vi "main.vi"() -> ()   [LabVIEW 2021]
uses:
  Global 1.vi
panel:
  in  "Boolean 2":bool
  in  "Tab Control":T1(tab)
  out "Curvas luz y temperatura":cluster{"Ramp Pattern":dbl[], dbl[]}[](graph)
  in  "Load":bool
  in  "Export":bool
  in  "Curva de Luz":path
  in  "Curva de Temperatura":path
  in  "Ruta Luz":path
  in  "Ruta Temperatura":path
  in  "Integrate":bool
  in  "X1 (s)":dbl
  in  "X2 (s)":dbl
  out "Resultado":dbl
  in  "Load 2":bool
  in  "Load 3":bool
  out "Curvas  Luz":cluster{"Ramp Pattern":dbl[], u32[]}[](graph)
  in  "Luz 4":path
  in  "Luz 3":path
  in  "Luz 2":path
  in  "Luz 1":path
  in  "Temperatura 4":path
  in  "Temperatura 3":path
  in  "Temperatura 2":path
  in  "Temperatura 1":path
  out "Curvas Temperatura":cluster{"Ramp Pattern":dbl[], u32[]}[](graph)
  # "Glow Curves\nAnalysis"
  # "Área de integración"
  # "Curvas de Temperatura"
  # "Curvas de Luz"
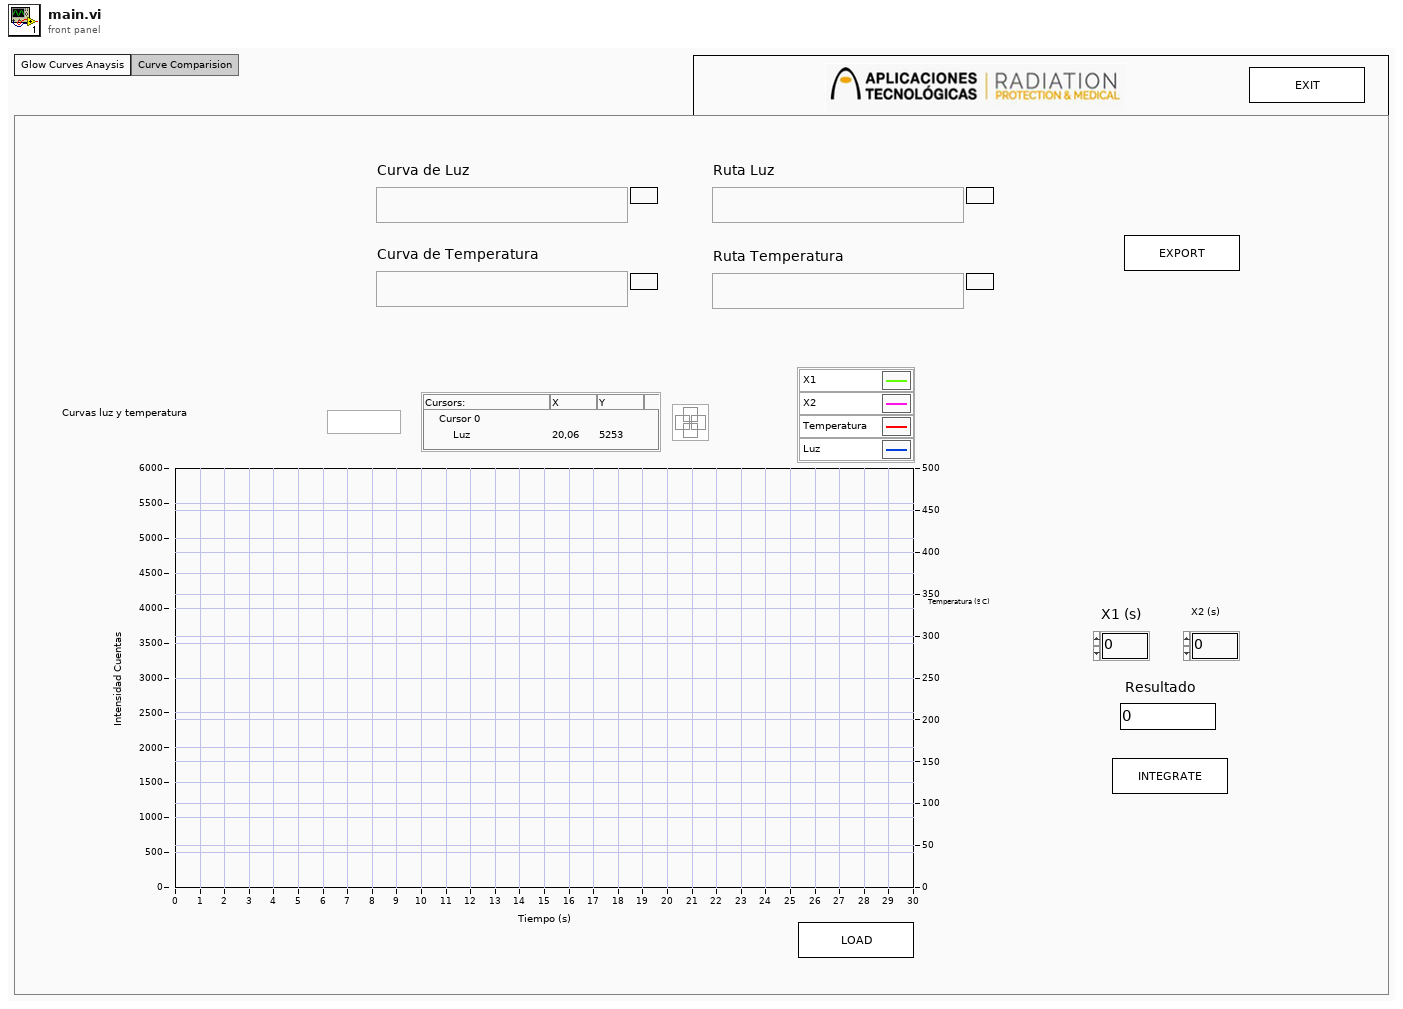
[diagram p1: front panel]
types:
  T1 = enum32{"Glow Curves Anaysis", "Curve Comparision"}
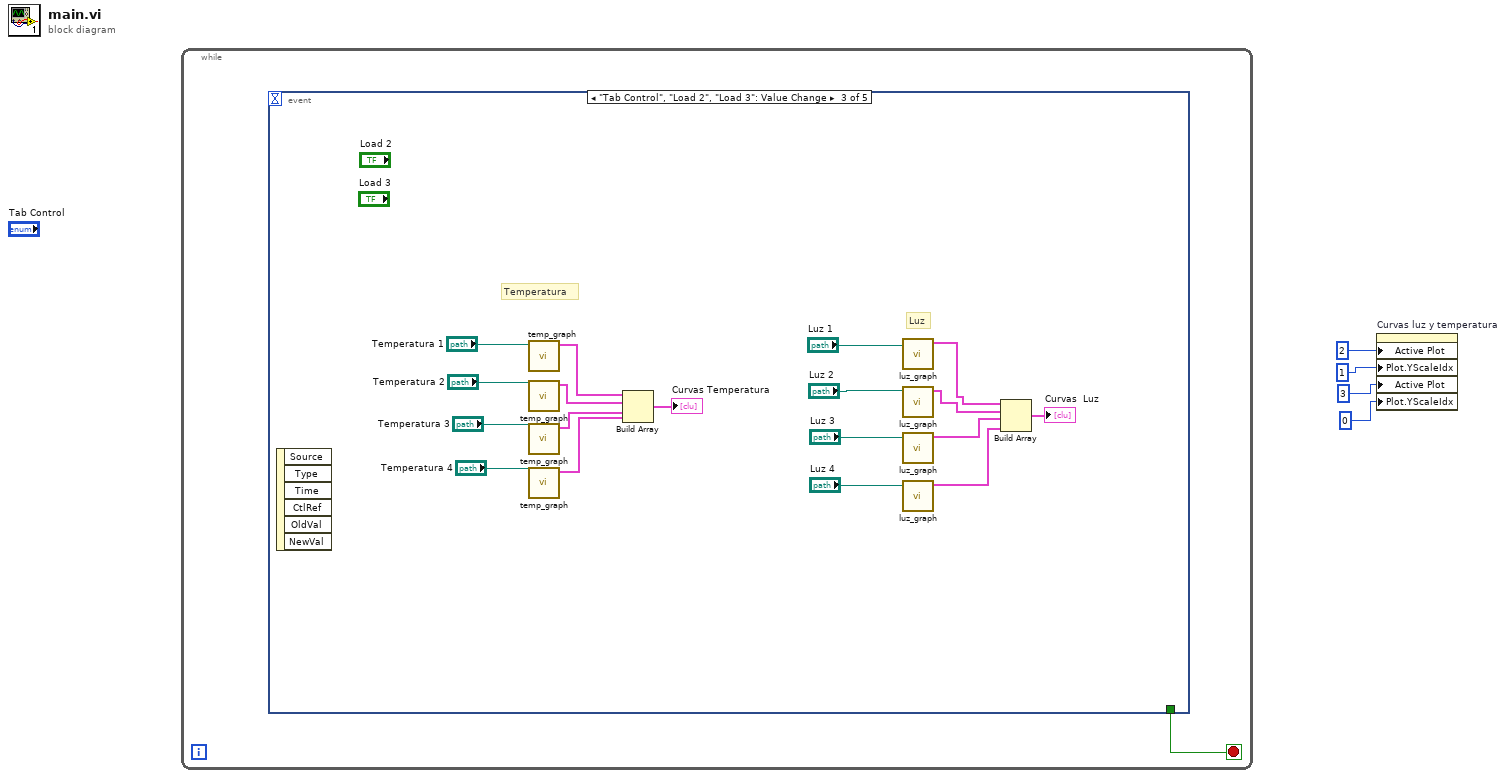
[diagram p0: block diagram]
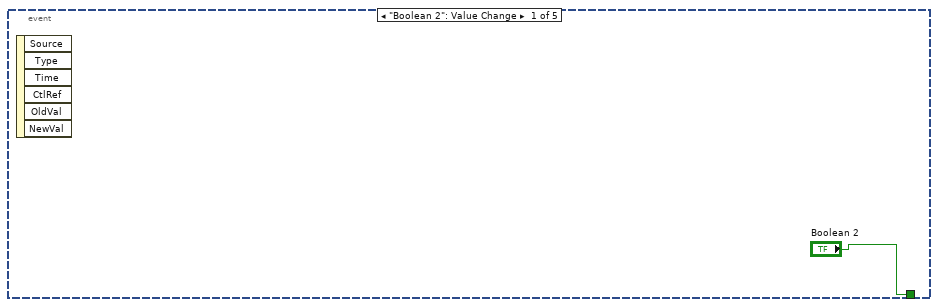
[diagram p2: hidden frame]
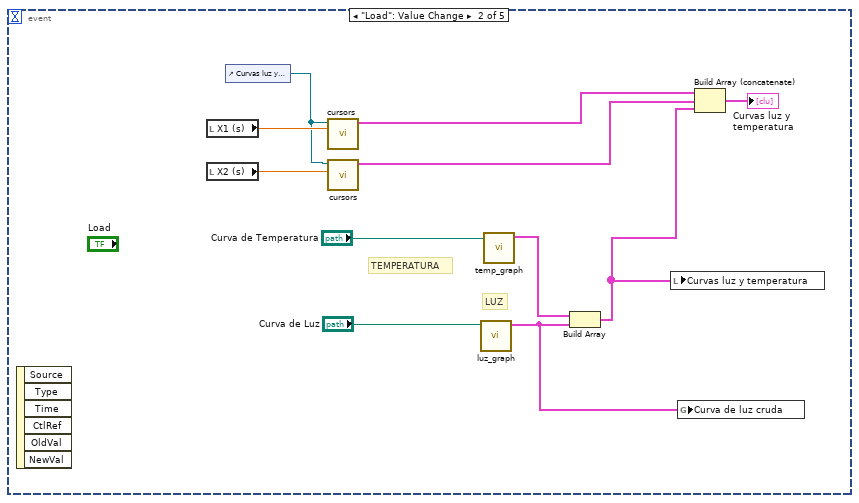
[diagram p3: hidden frame]
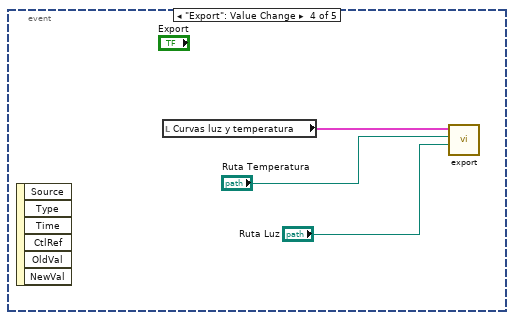
[diagram p4: hidden frame]
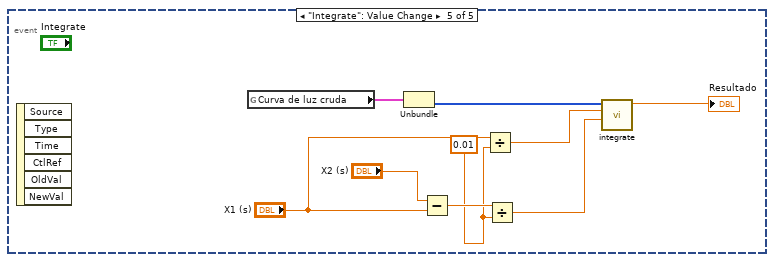
[diagram p5: hidden frame]
diagram:
  n1 = while {
    stop <- w5 stop-if-true
    n2 = event shown="[2] \"Tab Control\", \"Load 2\", \"Load 3\": Value Change" {
      selector: _ -> [_ _ _ _ _]
      dyn-events: _ -> [_ _ _ _ _]
      timeout: _ -> [_ _ _ _ _]
      tunnel: ["Boolean 2" _ _ _ _] -> w5
      event "Boolean 2": Value Change {
        n3 = event-data() -> ()  [unwired: 1 in, 6 out]
      }
      event "Load": Value Change {
        # "LUZ"
        # "TEMPERATURA"
        n4 = event-data() -> ()  [unwired: 1 in, 6 out]
        n5 = local read "X1 (s)"() -> (w12:dbl)
        n6 = local read "X2 (s)"() -> (w10:dbl)
        n7 = control-ref of="Curvas luz y temperatura"() -> (w11:refnum<vi>)
        n8 = call "cursors.vi"("X1 (s)"=w12, "XYGraph in"=w11) -> ("Cluster"=w9:cluster{dbl[], dbl[]})  [unwired: 9 in]
        n9 = call "cursors.vi"("X1 (s)"=w10, "XYGraph in"=w11) -> ("Cluster"=w8:cluster{dbl[], dbl[]})  [unwired: 9 in]
        n10 = call "luz_graph.vi"("file path (dialog if empty)"="Curva de Luz") -> ("Curva de luz"=w14:cluster{"Ramp Pattern":dbl[], u32[]})  [unwired: 10 in]
        n11 = call "temp_graph.vi"("file path (dialog if empty) in"="Curva de Temperatura") -> ("Curva de temperatura"=w17:cluster{"Ramp Pattern":dbl[], u32[]})  [unwired: 10 in]
        n12 = Build Array(w17, w14) -> (w13:cluster{"Ramp Pattern":dbl[], u32[]}[])
        n13 = local write "Curvas luz y temperatura"(w13) -> ()
        n14 = global write "Global 1.vi" "Curva de luz cruda"(w14) -> ()
        n15 = Build Array (concatenate)(w9, w8, w13) -> (→"Curvas luz y temperatura":cluster{"Ramp Pattern":dbl[], dbl[]}[])
      }
      event "Tab Control", "Load 2", "Load 3": Value Change {
        # "Luz"
        # "Temperatura"
        n16 = event-data() -> ()  [unwired: 1 in, 6 out]
        n17 = call "temp_graph.vi"("file path (dialog if empty) in"="Temperatura 1") -> ("Curva de temperatura"=w27:cluster{"Ramp Pattern":dbl[], u32[]})  [unwired: 10 in]
        n18 = call "temp_graph.vi"("file path (dialog if empty) in"="Temperatura 2") -> ("Curva de temperatura"=w26:cluster{"Ramp Pattern":dbl[], u32[]})  [unwired: 10 in]
        n19 = call "temp_graph.vi"("file path (dialog if empty) in"="Temperatura 3") -> ("Curva de temperatura"=w25:cluster{"Ramp Pattern":dbl[], u32[]})  [unwired: 10 in]
        n20 = call "temp_graph.vi"("file path (dialog if empty) in"="Temperatura 4") -> ("Curva de temperatura"=w24:cluster{"Ramp Pattern":dbl[], u32[]})  [unwired: 10 in]
        n21 = Build Array(w27, w26, w25, w24) -> (→"Curvas Temperatura":cluster{"Ramp Pattern":dbl[], u32[]}[])
        n22 = call "luz_graph.vi"("file path (dialog if empty)"="Luz 1") -> ("Curva de luz"=w23:cluster{"Ramp Pattern":dbl[], u32[]})  [unwired: 10 in]
        n23 = call "luz_graph.vi"("file path (dialog if empty)"="Luz 2") -> ("Curva de luz"=w22:cluster{"Ramp Pattern":dbl[], u32[]})  [unwired: 10 in]
        n24 = call "luz_graph.vi"("file path (dialog if empty)"="Luz 3") -> ("Curva de luz"=w21:cluster{"Ramp Pattern":dbl[], u32[]})  [unwired: 10 in]
        n25 = call "luz_graph.vi"("file path (dialog if empty)"="Luz 4") -> ("Curva de luz"=w20:cluster{"Ramp Pattern":dbl[], u32[]})  [unwired: 10 in]
        n26 = Build Array(w23, w22, w21, w20) -> (→"Curvas  Luz":cluster{"Ramp Pattern":dbl[], u32[]}[])
      }
      event "Export": Value Change {
        n27 = event-data() -> ()  [unwired: 1 in, 6 out]
        n28 = local read "Curvas luz y temperatura"() -> (w38:cluster{"Ramp Pattern":dbl[], dbl[]}[])
        n29 = call "export.vi"("Ruta luz"="Ruta Luz", "Ruta Temp"="Ruta Temperatura", "Curva de Luz y Temperatura 3"=w38) -> ()  [unwired: 9 in]
      }
      event "Integrate": Value Change {
        w43 = 0.01 ("y")
        n30 = event-data() -> ()  [unwired: 1 in, 6 out]
        n31 = global read "Global 1.vi" "Curva de luz cruda"() -> (w47:cluster{"Ramp Pattern":dbl[], u32[]})
        n32 = Unbundle(w47) -> (w46:u32[])  [unwired: 1 out]
        n33 = Subtract(x="X2 (s)", y="X1 (s)") -> (x-y=w44:dbl)
        n34 = Divide(x="X1 (s)", y=w43) -> (x/y=w40:dbl)
        n35 = Divide(x=w44, y=w43) -> (x/y=w41:dbl)
        n36 = call "integrate.vi"("Longitud"=w41, "inicio"=w40, "Array"=w46) -> ("result"=→"Resultado":dbl)  [unwired: 8 in]
      }
    }
  }
  n37 = property on="Curvas luz y temperatura" class="XYGraph (strict)"("Active Plot"=u32 2, "Plot.YScaleIdx"=u32 1 ("Plot.Y Scale Index"), "Active Plot"=u32 3, "Plot.YScaleIdx"=u32 0 ("Plot.Y Scale Index")) -> ()  [unwired: 2 in, 2 out]
